vi "Финал.vi"() -> ()   [LabVIEW 2017]
panel:
  in  "C":bool
  out "Cluster 2":T1
  out "Cluster":T1
  in  "adrB":cluster{"h1":bool, "h0":bool}
  in  "adrA":cluster{"h1":bool, "h0":bool}
  in  "WR":bool
  in  "R":bool
  in  "4 final":T2
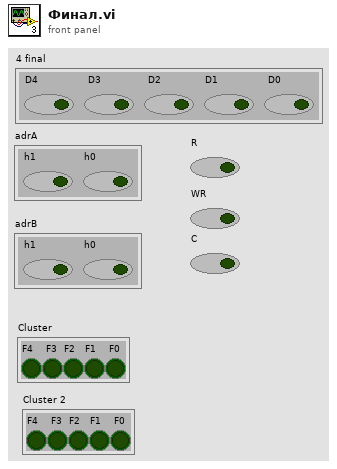
[diagram p1: front panel]
types:
  T1 = cluster{"F4":bool, " F3":bool, "F2":bool, "F1":bool, " F0":bool}
  T2 = cluster{"D4":bool, " D3":bool, " D2":bool, "D1":bool, " D0":bool}
  T3 = cluster{"c1":bool, "c2":bool, "c3":bool, "c4":bool}
  T4 = cluster{"Boolean":bool, "Boolean 2":bool, "Boolean 3":bool, "Boolean 4":bool, "Boolean 5":bool}
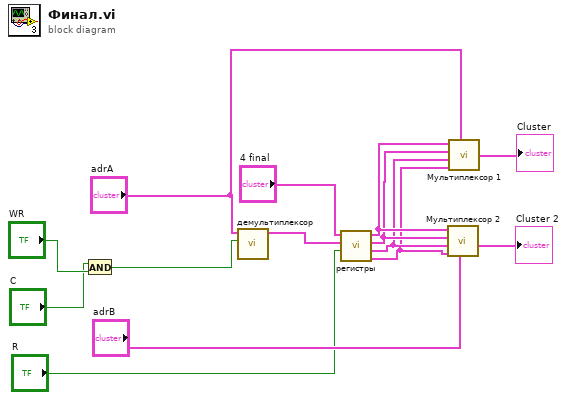
[diagram p0: block diagram]
diagram:
  n1 = And(x="C", y="WR") -> (x .and. y?=w1:bool)
  n2 = call "демультиплексор.vi"("C / WR"=w1, "adrA"="adrA") -> ("Cluster"=w3:T3)  [unwired: 5 in]
  n3 = call "регистры.vi"("R"="R", "Cluster"=w3, "4"="4 final") -> ("4"=w5:T4, "3"=w6:T4, "2"=w7:T4, "1"=w8:T4)  [unwired: 1 in]
  n4 = call "Мультиплексор 2.vi"("1"=w8, "2"=w7, "3"=w6, "4"=w5, "adrB"="adrB") -> ("Cluster"=→"Cluster 2":T1)
  n5 = call "Мультиплексор 1.vi"("1"=w8, "2"=w7, "3"=w6, "4"=w5, "adrA"="adrA") -> ("Cluster"=→"Cluster":T1)
